vi "Simulation Data_Global.vi"() -> ()   [LabVIEW 2013, in "Simulation.lvlib"]
uses:
  Simulation.lvlib
panel:
  in  "Result":dbl
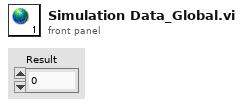
[diagram p1: front panel]
diagram:
